vi "DeppDisable.vi"(8 "Error In":errorcluster, 11 "Device Handle":u32) -> (0 "Error Out":errorcluster, 3 "Device Handle":u32)   [LabVIEW 2011, in "LVH-Adept.lvlib" / "DEPP.lvlib"]
uses:
  <vilib>/LabVIEW Hacker/Adept/Private/DEPP/DEPP.lvlib
  <vilib>/LabVIEW Hacker/Adept/Private/DEPP/Private/Type Defs/Error.ctl
  <vilib>/LabVIEW Hacker/Adept/Private/Resources/depp.dll
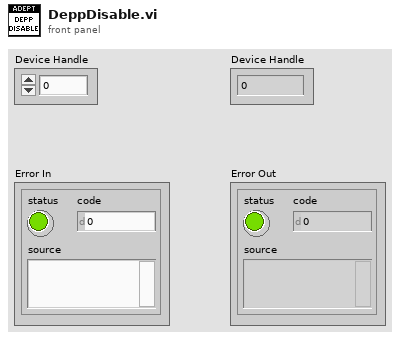
[diagram p1: front panel]
types:
  T1 = typedef "LVH-Adept.lvlib/DEPP.lvlib/Error.ctl" = enum16{"Unknown", "Enable", "Get Register", "Get Register Repeat", "Get Register Set", "Put Register", "Put Register Repeat", "Put Register Set", "Disable", "Set Pair Size"}
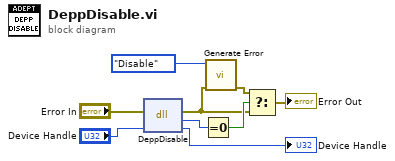
[diagram p0: block diagram]
diagram:
  n1 = dll-call lib="C:/Program Files (x86)/National Instruments/LabVIEW 2011/vi.lib/LabVIEW Hacker/Adept/Private/Resources/depp.dll" fn="DeppDisable"(error in="Error In", "hif"="Device Handle") -> (error out=w1:errorcluster, "Success"=w8:u32, "hif"=→"Device Handle":u32)  [unwired: 2 in, 1 out]
  n2 = Equal To 0?(x=w8) -> (x = 0?=w7:bool)
  n3 = call <vilib>:"Generate Error.vi"("Error In"=w1, "DEPP Error"=Error."Disable") -> ("Error Out"=w2:errorcluster)  [unwired: 9 in]
  n4 = Select(t=w2, s=w7, f=w1) -> (s? t:f=→"Error Out":errorcluster)
